vi "PicoScope4000aWrapSettings.vi"(7 "Unit Info":T1, 8 "error in (no error)":errorcluster, 9 "Enabled array":i16[](array[numeric]), 11 "Handle In":i16) -> (0 "error out":errorcluster, 3 "Handle Out":i16)   [LabVIEW 2010]
uses:
  ps4000aWrap.dll
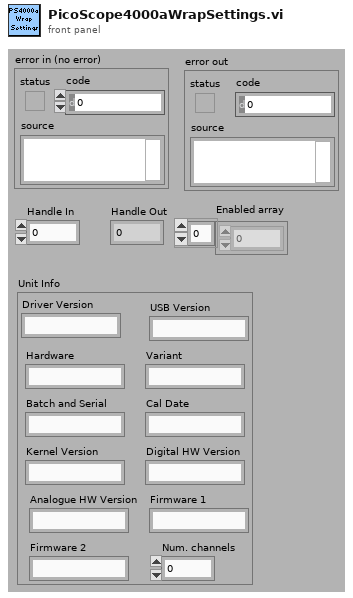
[diagram p1: front panel]
types:
  T1 = cluster{"Driver Version":string, "USB Version":string, "Hardware":string, "Variant":string, "Batch and Serial":string, "Cal Date":string, "Kernel Version":string, "Digital HW Version":string, "Analogue HW Version":string, "Firmware 1":string, "Firmware 2":string, "Num. channels":i16}
  T2 = cluster{"status":bool, "code":u32, "source":string}
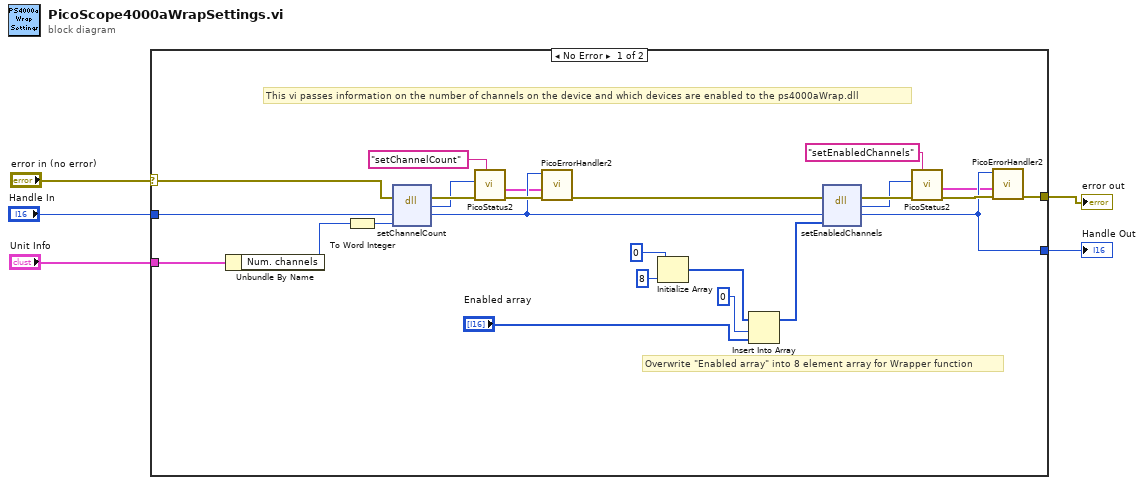
[diagram p0: block diagram]
diagram:
  n1 = case shown="No Error" "error in (no error)" {
    selector: "error in (no error)" -> [w8 w32]
    tunnel: "Handle In" -> [w30 w31]
    tunnel: [w19 w32] -> w4
    tunnel: [w18 w31] -> w3
    tunnel: "Unit Info" -> [w16 _]
    frame No Error {
      # "Overwrite \"Enabled array\" into 8 element array for Wrapper function"
      # "This vi passes information on the number of channels on the device and which devices are enabled to the ps4000aWrap.dll"
      n2 = Unbundle By Name(w16) -> ("Num. channels"=w15:i16)
      n3 = To Word Integer(number=w15) -> (16bit integer=w17:i16)
      n4 = dll-call lib="ps4000aWrap.dll" fn="setChannelCount"(error in=w8, "handle"=w30, "channelCount"=w17) -> (error out=w28:errorcluster, "PICO_STATUS"=w27:u32, "handle"=w24:i16)  [unwired: 3 in, 1 out]
      n5 = call "PicoStatus2.vi"("PICO source"="setChannelCount" ("source"), "Error in"=w28, "PICO STATUS"=w27) -> ("error out"=w29:errorcluster, "PICO_STATUS out"=w7:T2)  [unwired: 5 in]
      n6 = call "PicoErrorHandler2.vi"("error in (no error)"=w29, "PICO_STATUS in"=w7, "handle In"=w24) -> ("error out"=w25:errorcluster)  [unwired: 8 in]
      n7 = Initialize Array(i16 0 ("element"), 8 ("dimension size")) -> (w12:i16[])
      n8 = Insert Into Array(array=w12, index=0, new element="Enabled array") -> (w9:i16[])
      n9 = dll-call lib="ps4000aWrap.dll" fn="setEnabledChannels"(error in=w25, "handle"=w24, "enabledChannels"=w9) -> (error out=w21:errorcluster, "PICO_STATUS"=w20:u32, "handle"=w18:i16)  [unwired: 3 in, 1 out]
      n10 = call "PicoStatus2.vi"("PICO source"="setEnabledChannels" ("source"), "Error in"=w21, "PICO STATUS"=w20) -> ("error out"=w23:errorcluster, "PICO_STATUS out"=w6:T2)  [unwired: 5 in]
      n11 = call "PicoErrorHandler2.vi"("error in (no error)"=w23, "PICO_STATUS in"=w6, "handle In"=w18) -> ("error out"=w19:errorcluster)  [unwired: 8 in]
    }
    frame Error {
    }
  }
  "Handle Out" <- w3
  "error out" <- w4
